vi "strain sensor program.vi"() -> ()   [LabVIEW 2016]
uses:
  Program Files (x86)/National Instruments/LabVIEW 2017/instr.lib/Keithley 2000/Keithley 2000.lvlib
  Program Files (x86)/National Instruments/LabVIEW 2017/instr.lib/Keithley 2000/Public/Configure/Configure 2 Wire Resistance.vi
  Program Files (x86)/National Instruments/LabVIEW 2017/instr.lib/Keithley 2000/Public/Configure/Configure DC Current.vi
  Program Files (x86)/National Instruments/LabVIEW 2017/instr.lib/Keithley 2000/Public/Configure/Configure AC Current.vi
  Program Files (x86)/National Instruments/LabVIEW 2017/instr.lib/Keithley 2000/Public/Configure/Configure DC Volts.vi
  Program Files (x86)/National Instruments/LabVIEW 2017/instr.lib/Keithley 2000/Public/Configure/Configure AC Volts.vi
  Program Files (x86)/National Instruments/LabVIEW 2017/instr.lib/Keithley 2000/Public/Configure/Configure 4 Wire Resistance.vi
  <vilib>/Utility/file.llb/Write To Spreadsheet File (DBL).vi
panel:
  out "point numbers 2":i32
  out "Measurement 2":dbl
  out "Units 2":string
  out "Speed(X) 2":i32
  out "Position(X) 2":i32
  out "XY 그래프 2":cluster{dbl[], dbl[]}(graph)
  in  "?":bool
  in  "?":u16(ring) items=["+X", "-X", "+Y", "-Y"]
  out "Units":string
  out "Measurement":dbl
  in  "Function (0: DC Volts)":u16(ring)=4 items=["DC Volts", "AC Volts", "DC Current", "AC Current", "2-Wire Resistance", "4-Wire Resistance"]
  in  "VISA resource name":refnum<visa-resource-name>="GPIB0::16::INSTR"
  out "XY 그래프":cluster{dbl[], dbl[]}(graph)
  in  "file path (dialog if empty)":path
  out "Position(X)":i32
  out "Speed(X)":i32
  in  "Start":bool
  out "point numbers":i32
  in  "?":bool
  in  "?":u16(ring) items=["X", "Y"]
  in  "Set Speed":i32
  out "Read Speed":u32
  in  "Drive Speed Number":u16(ring) items=["Drive Speed 1", "Drive Speed 2", "Drive Speed 3", "Drive Speed 4"]
  in  "Drive speed Set":bool
  in  "Drive Speed Number":u16(ring) items=["Drive Speed 1", "Drive Speed 2", "Drive Speed 3", "Drive Speed 4"]
  in  "Axis":u16(ring) items=["X", "Y"]
  out "Speed":u32=1000
  in  "Speed Set":bool
  in  "AXIS":u16(ring)=1 items=["X", "Y"]
  in  "SPEED(1~4)":string="1"
  in  "x - axis start point (cm)":dbl
  out "baud rate output":refnum<visa-resource-name>
  in  "x - axis increment(cm)":dbl
  in  "baud rate (9600)":u32=9600
  in  "Port set":refnum<visa-resource-name>="COM3"
  in  "x - axis end point (cm)":dbl=10.0
  in  "?":bool
  # "Motor Control"
  # "DRIVE SPEED READ"
  # "DRIVE SPEED SELECT"
  # "DRIVE SPEED SET"
  # "Plot : Ohm-cm"
  # "POSITION & SPEED READ"
  # "Multimeter"
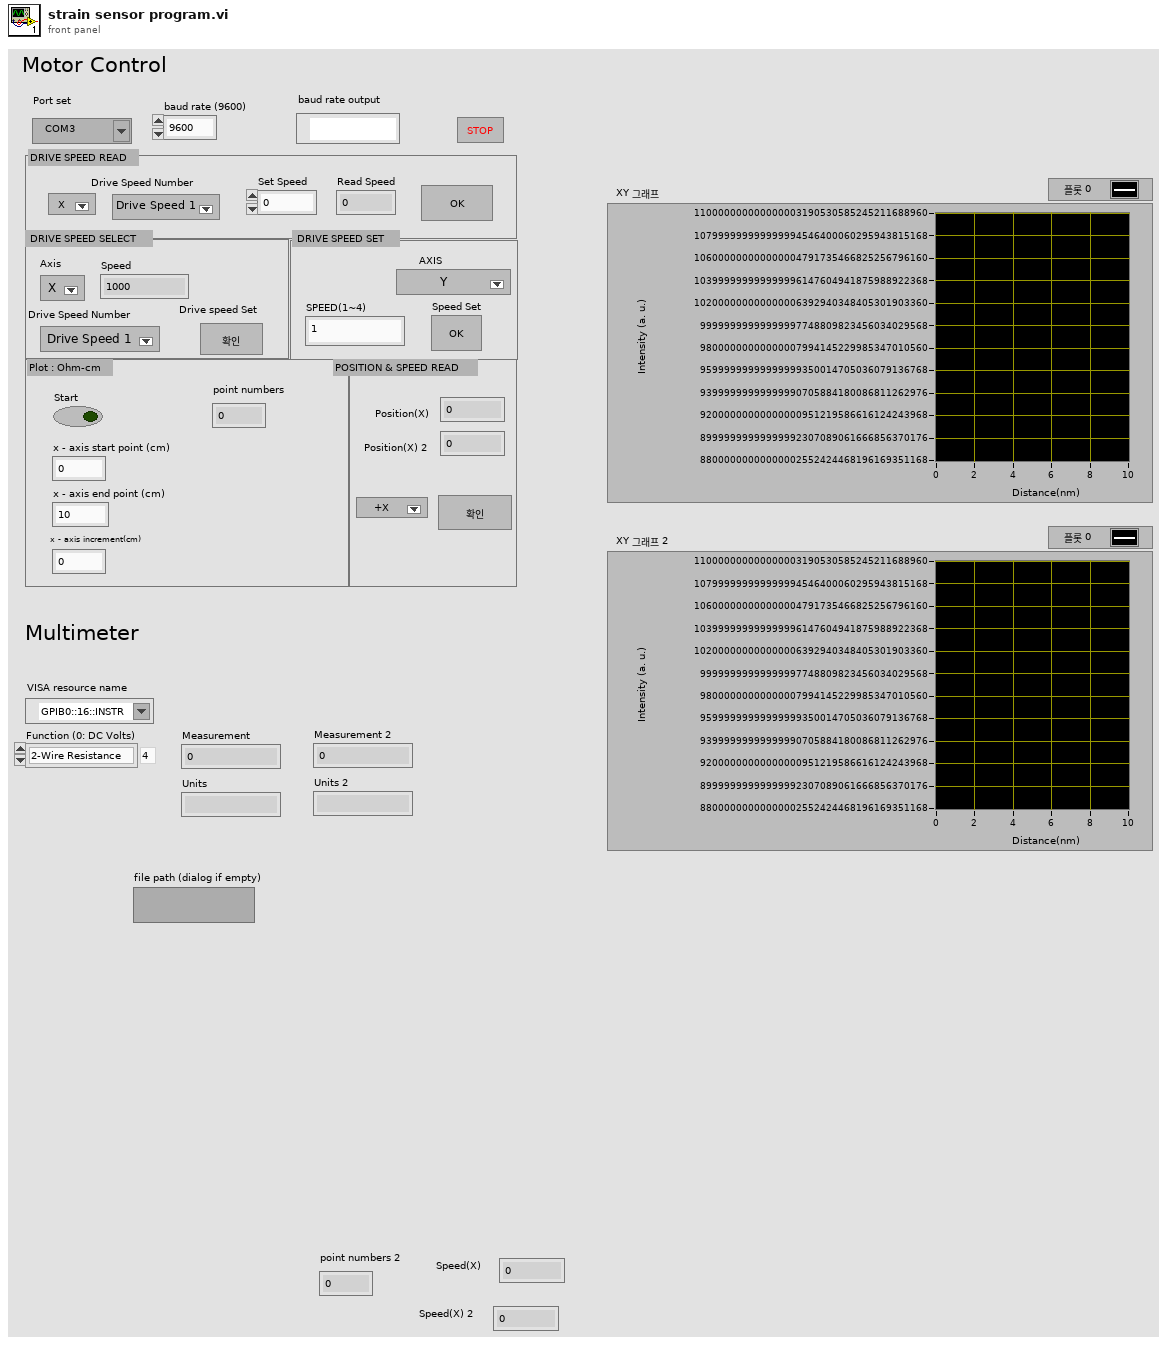
[diagram p1: front panel]
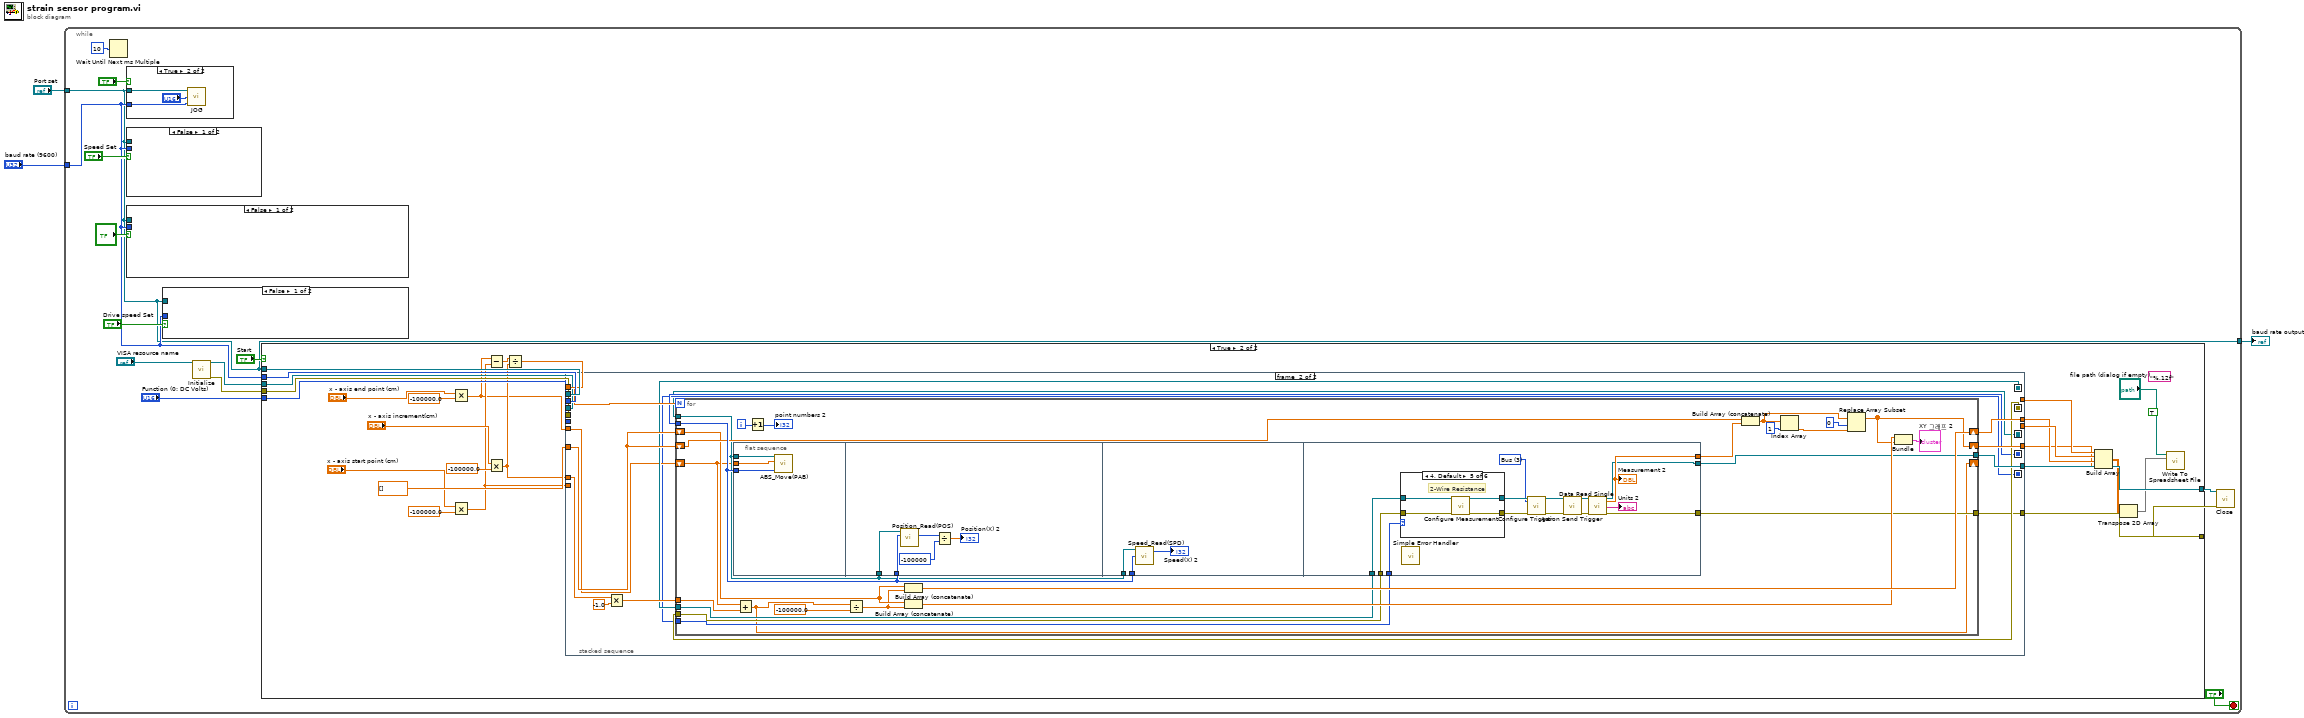
[diagram p0: block diagram]
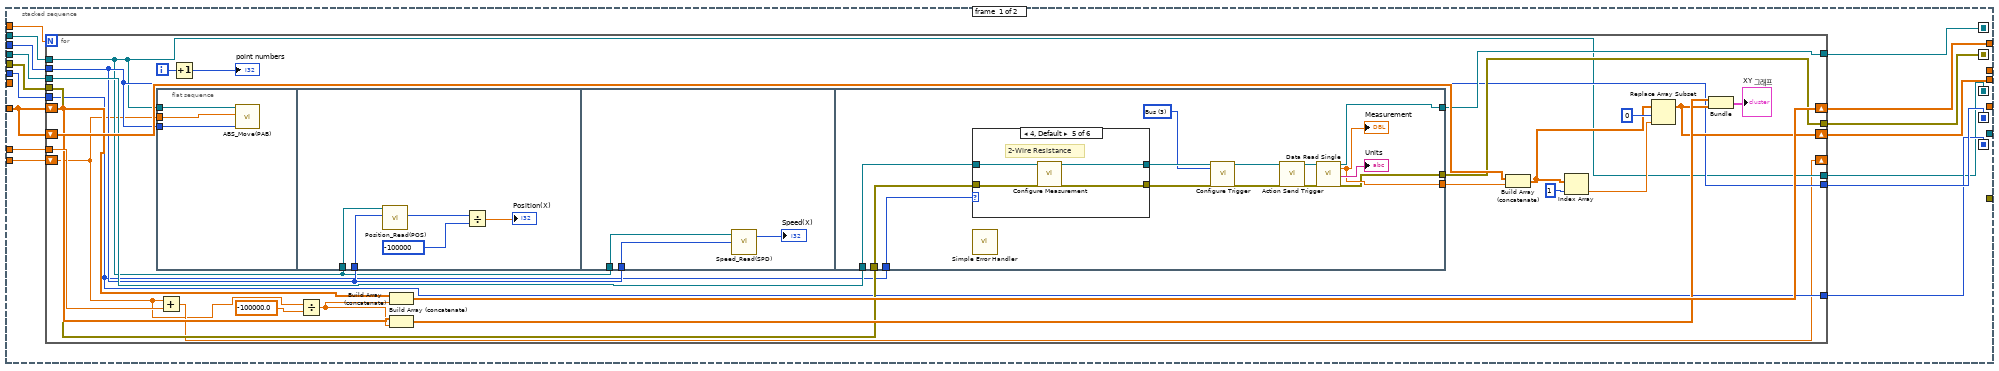
[diagram p4: hidden frame]
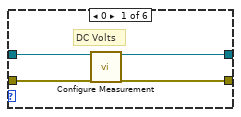
[diagram p5: hidden frame]
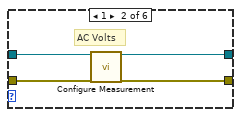
[diagram p6: hidden frame]
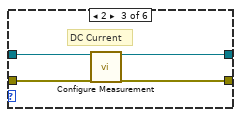
[diagram p7: hidden frame]
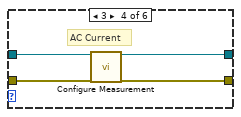
[diagram p8: hidden frame]
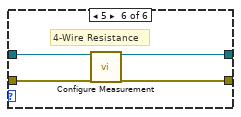
[diagram p9: hidden frame]
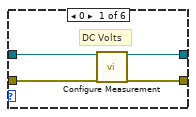
[diagram p10: hidden frame]
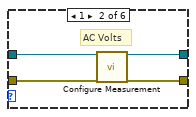
[diagram p11: hidden frame]
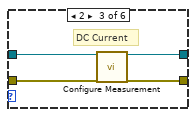
[diagram p12: hidden frame]
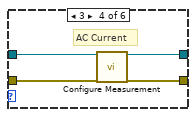
[diagram p13: hidden frame]
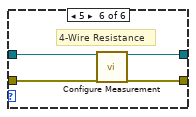
[diagram p14: hidden frame]
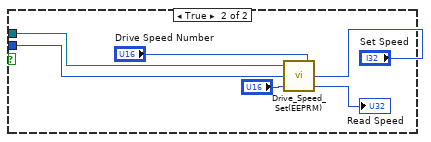
[diagram p15: hidden frame]
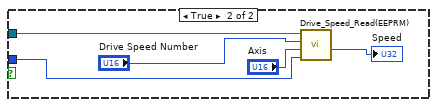
[diagram p16: hidden frame]
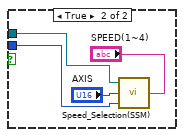
[diagram p17: hidden frame]
diagram:
  n1 = while {
    tunnel: "Port set" -> [w4]
    tunnel: "baud rate (9600)" -> [w5]
    tunnel: [w4] -> w1
    stop <- "?" stop-if-true
    n2 = Wait Until Next ms Multiple(millisecond multiple=u32 10 ("ms 배수")) -> ()  [unwired: 1 out]
    n3 = case shown="True" "?" {
      tunnel: w4 -> [_ w21]
      tunnel: w5 -> [_ w20]
      frame False {
      }
      frame True {
        n4 = call "JOG.vi"("baud rate (9600)"=w20, "AXIS"="?", "Port"=w21) -> ()  [unwired: 2 out]
      }
    }
    n5 = case shown="False" "Speed Set" {
      tunnel: w4 -> [_ w241]
      tunnel: w5 -> [_ w240]
      frame False {
      }
      frame True {
        n6 = call "Speed_Selection(SSM).vi"("SPEED(1~4)"="SPEED(1~4)", "baud rate (9600)"=w240, "AXIS"="AXIS", "Port"=w241) -> ()  [unwired: 2 out]
      }
    }
    n7 = case shown="False" "?" {
      tunnel: w4 -> [_ w232]
      tunnel: w5 -> [_ w227]
      frame False {
      }
      frame True {
        n8 = call "Drive_Speed_Set(EEPRM).vi"("Set Speed"="Set Speed", "Drive Speed Number"="Drive Speed Number", "Axis"="?", "baud rate (9600)"=w227, "Port"=w232) -> ("Read Speed"=→"Read Speed":u32)
      }
    }
    n9 = case shown="False" "Drive speed Set" {
      tunnel: w4 -> [_ w237]
      tunnel: w5 -> [_ w233]
      frame False {
      }
      frame True {
        n10 = call "Drive_Speed_Read(EEPRM).vi"("baud rate (9600)"=w233, "Axis"="Axis", "Drive Speed Number"="Drive Speed Number", "Port"=w237) -> ("Spped"=→"Speed":u32)  [unwired: 1 in, 3 out]
      }
    }
    n11 = call "Initialize.vi"("VISA resource name"="VISA resource name") -> ("VISA resource name out"=w10:refnum<visa-resource-name>, "error out"=w9:errorcluster)  [unwired: 17 in]
    n12 = case shown="True" "Start" {
      tunnel: w4 -> [_ w47]
      tunnel: w5 -> [_ w46]
      tunnel: "Function (0: DC Volts)" -> [_ w40]
      tunnel: w10 -> [_ w39]
      tunnel: w9 -> [_ w38]
      tunnel: [_ w37] -> w8
      tunnel: [_ w36] -> w7
      frame False {
      }
      frame True {
        (unwired) "%.12f" ("format (%.3f)")
        (unwired) TRUE
        n13 = Multiply(x="x - axis end point (cm)", y=-100000.0) -> (x*y=w27:dbl)
        n14 = Multiply(x="x - axis start point (cm)", y=-100000.0) -> (x*y=w28:dbl)
        n15 = Subtract(x=w27, y=w28) -> (x-y=w45:dbl)
        n16 = Multiply(x="x - axis increment(cm)", y=-100000.0) -> (x*y=w31:dbl)
        n17 = Divide(x=w45, y=w31) -> (x/y=w44:dbl)
        n18 = stacked-sequence {
          seq-local: [w52 _] -> [_ w144]
          seq-local: [w51 _] -> [_ w143]
          seq-local: [w50 _] -> [_ w140]
          seq-local: [w49 _] -> [_ w139]
          seq-local: [w48 _] -> [_ w138]
          tunnel: w47 -> [w63 _]
          tunnel: w46 -> [w62 _]
          tunnel: w44 -> [w61 w151]
          tunnel: dbl[] [] -> [w60 w152]
          tunnel: [w59 _] -> w42
          tunnel: [w58 _] -> w41
          tunnel: w40 -> [w57 _]
          tunnel: w39 -> [w56 _]
          tunnel: w38 -> [w55 _]
          tunnel: [_ w145] -> w37
          tunnel: [_ w142] -> w36
          tunnel: w31 -> [w54 w149]
          tunnel: w28 -> [w53 _]
          tunnel: [_ w147] -> w25
          tunnel: [_ w146] -> w24
          tunnel: w27 -> [_ w141]
          frame #0 {
            n19 = for {
              N: w61 -> [_]
              tunnel: w54 -> [w86]
              shift-right: [w65] -> _
              shift-left: w53 -> [w64]
              tunnel: w63 -> [w66]
              tunnel: w62 -> [w68]
              shift-right: [w84] -> w59
              shift-left: w60 -> [w81]
              shift-right: [w70] -> w58
              shift-left: w60 -> [w85]
              tunnel: w57 -> [w67]
              tunnel: w56 -> [w80]
              tunnel: w55 -> [w79]
              tunnel: [w78] -> w52
              tunnel: [w77] -> w51
              tunnel: [w68] -> w50
              tunnel: [w67] -> w49
              tunnel: [w66] -> w48
              i -> [w88]
              n20 = flat-sequence {
                tunnel: w68 -> [w91]
                tunnel: w66 -> [w90]
                tunnel: w64 -> [w89]
                tunnel: w68 -> [w96]
                tunnel: w66 -> [w95]
                tunnel: w68 -> [w98]
                tunnel: w66 -> [w97]
                tunnel: [w105] -> w82
                tunnel: w67 -> [w104]
                tunnel: w80 -> [w103]
                tunnel: w79 -> [w102]
                tunnel: [w101] -> w78
                tunnel: [w100] -> w77
                frame #0 {
                  n21 = call "ABS_Move(PAB).vi"("baud rate (9600)"=w91, "X Position(ABS)"=w89, "Port"=w90) -> ()  [unwired: 3 in, 3 out]
                }
                frame #1 {
                  n22 = call "Position_Read(POS).vi"("baud rate (9600)"=w96, "Port"=w95) -> ("Position(X)"=w93:i32)  [unwired: 2 in, 4 out]
                  n23 = Divide(x=w93, y=-100000) -> (x/y=→"Position(X)":dbl)
                }
                frame #2 {
                  n24 = call "Speed_Read(SPD).vi"("baud rate (9600)"=w98, "Port"=w97) -> ("Speed(X)"=→"Speed(X)":i32)  [unwired: 1 in, 2 out]
                }
                frame #3 {
                  w110 = u16 3 items=["Immediate", "Timer", "Manual", "Bus", "External"] ("Source (0: Immediate)")
                  n25 = case shown="4, Default" w104 {
                    tunnel: w102 -> [w117 w121 w125 w129 w133 w137]
                    tunnel: w103 -> [w116 w120 w124 w128 w132 w136]
                    tunnel: [w115 w119 w123 w127 w131 w135] -> w113
                    tunnel: [w114 w118 w122 w126 w130 w134] -> w112
                    frame 0 {
                      # "DC Volts"
                      n26 = call-poly "Configure Measurement.vi"("VISA resource name"=w116, "error in (no error)"=w117) -> ("VISA resource name out"=w114:refnum<visa-resource-name>, "error out"=w115:errorcluster)  [unwired: 16 in]
                    }
                    frame 1 {
                      # "AC Volts"
                      n27 = call-poly "Configure Measurement.vi"("VISA resource name"=w120, "error in (no error)"=w121) -> ("VISA resource name out"=w118:refnum<visa-resource-name>, "error out"=w119:errorcluster)  [unwired: 16 in]
                    }
                    frame 2 {
                      # "DC Current"
                      n28 = call-poly "Configure Measurement.vi"("VISA resource name"=w124, "error in (no error)"=w125) -> ("VISA resource name out"=w122:refnum<visa-resource-name>, "error out"=w123:errorcluster)  [unwired: 16 in]
                    }
                    frame 3 {
                      # "AC Current"
                      n29 = call-poly "Configure Measurement.vi"("VISA resource name"=w128, "error in (no error)"=w129) -> ("VISA resource name out"=w126:refnum<visa-resource-name>, "error out"=w127:errorcluster)  [unwired: 16 in]
                    }
                    frame 4, Default {
                      # "2-Wire Resistance"
                      n30 = call-poly "Configure Measurement.vi"("VISA resource name"=w132, "error in (no error)"=w133) -> ("VISA resource name out"=w130:refnum<visa-resource-name>, "error out"=w131:errorcluster)  [unwired: 16 in]
                    }
                    frame 5 {
                      # "4-Wire Resistance"
                      n31 = call-poly "Configure Measurement.vi"("VISA resource name"=w136, "error in (no error)"=w137) -> ("VISA resource name out"=w134:refnum<visa-resource-name>, "error out"=w135:errorcluster)  [unwired: 16 in]
                    }
                  }
                  n32 = call <vilib>:"Simple Error Handler.vi"() -> ()  [unwired: 5 in, 5 out]
                  n33 = call "Configure Trigger.vi"("VISA resource name"=w112, "Source (0: Immediate)"=w110, "error in (no error)"=w113) -> ("VISA resource name out"=w109:refnum<visa-resource-name>, "error out"=w108:errorcluster)  [unwired: 15 in]
                  n34 = call "Action Send Trigger.vi"("VISA resource name"=w109, "error in (no error)"=w108) -> ("VISA resource name out"=w106:refnum<visa-resource-name>, "error out"=w107:errorcluster)  [unwired: 16 in]
                  n35 = call "Data Read Single.vi"("VISA resource name"=w106, "error in (no error)"=w107) -> ("VISA resource name out"=w101:refnum<visa-resource-name>, "Measurement"=w105:dbl, "Units"=→"Units":string, "error out"=w100:errorcluster)  [unwired: 13 in, 1 out]
                  "Measurement" <- w105
                }
              }
              n36 = Add(x=w64, y=w86) -> (x+y=w65:dbl)
              n37 = Increment(x=w88) -> (x+1=→"point numbers":i32)
              n38 = Divide(x=w64, y=-100000.0) -> (x/y=w72:dbl)
              n39 = Build Array (concatenate)(w81, w72) -> (w84:dbl[])
              n40 = Build Array (concatenate)(w81, w72) -> (w83:dbl[])
              n41 = Build Array (concatenate)(w85, w82) -> (w71:dbl[])
              n42 = Index Array(array=w71, index=1) -> (element=w74:dbl)
              n43 = Replace Array Subset(array=w71, new element=w74, index=0) -> (w70:dbl[])
              n44 = Bundle(w83, w70) -> (→"XY 그래프":cluster{dbl[], dbl[]})  [unwired: 1 in]
            }
          }
          frame #1 {
            n45 = Multiply(x=w149, y=-1.0) -> (x*y=w148:dbl)
            n46 = for {
              N: w151 -> [_]
              tunnel: w148 -> [w174]
              shift-right: [w158] -> _
              shift-left: w141 -> [w153]
              tunnel: w138 -> [w154]
              tunnel: w140 -> [w175]
              shift-right: [w172] -> w147
              shift-left: w152 -> [w169]
              shift-right: [w156] -> w146
              shift-left: w152 -> [w173]
              tunnel: w139 -> [w168]
              tunnel: w144 -> [w167]
              tunnel: w143 -> [w166]
              tunnel: [w165] -> w145
              tunnel: [w164] -> w142
              i -> [w177]
              n47 = flat-sequence {
                tunnel: w175 -> [w180]
                tunnel: w154 -> [w179]
                tunnel: w153 -> [w178]
                tunnel: w175 -> [w185]
                tunnel: w154 -> [w184]
                tunnel: w175 -> [w187]
                tunnel: w154 -> [w186]
                tunnel: [w194] -> w170
                tunnel: w168 -> [w193]
                tunnel: w167 -> [w192]
                tunnel: w166 -> [w191]
                tunnel: [w190] -> w165
                tunnel: [w189] -> w164
                frame #0 {
                  n48 = call "ABS_Move(PAB).vi"("baud rate (9600)"=w180, "X Position(ABS)"=w178, "Port"=w179) -> ()  [unwired: 3 in, 3 out]
                }
                frame #1 {
                  n49 = call "Position_Read(POS).vi"("baud rate (9600)"=w185, "Port"=w184) -> ("Position(X)"=w182:i32)  [unwired: 2 in, 4 out]
                  n50 = Divide(x=w182, y=-100000) -> (x/y=→"Position(X) 2":dbl)
                }
                frame #2 {
                  n51 = call "Speed_Read(SPD).vi"("baud rate (9600)"=w187, "Port"=w186) -> ("Speed(X)"=→"Speed(X) 2":i32)  [unwired: 1 in, 2 out]
                }
                frame #3 {
                  w199 = u16 3 items=["Immediate", "Timer", "Manual", "Bus", "External"] ("Source (0: Immediate)")
                  n52 = case shown="4, Default" w193 {
                    tunnel: w191 -> [w206 w210 w214 w218 w222 w226]
                    tunnel: w192 -> [w205 w209 w213 w217 w221 w225]
                    tunnel: [w204 w208 w212 w216 w220 w224] -> w202
                    tunnel: [w203 w207 w211 w215 w219 w223] -> w201
                    frame 0 {
                      # "DC Volts"
                      n53 = call-poly "Configure Measurement.vi"("VISA resource name"=w205, "error in (no error)"=w206) -> ("VISA resource name out"=w203:refnum<visa-resource-name>, "error out"=w204:errorcluster)  [unwired: 16 in]
                    }
                    frame 1 {
                      # "AC Volts"
                      n54 = call-poly "Configure Measurement.vi"("VISA resource name"=w209, "error in (no error)"=w210) -> ("VISA resource name out"=w207:refnum<visa-resource-name>, "error out"=w208:errorcluster)  [unwired: 16 in]
                    }
                    frame 2 {
                      # "DC Current"
                      n55 = call-poly "Configure Measurement.vi"("VISA resource name"=w213, "error in (no error)"=w214) -> ("VISA resource name out"=w211:refnum<visa-resource-name>, "error out"=w212:errorcluster)  [unwired: 16 in]
                    }
                    frame 3 {
                      # "AC Current"
                      n56 = call-poly "Configure Measurement.vi"("VISA resource name"=w217, "error in (no error)"=w218) -> ("VISA resource name out"=w215:refnum<visa-resource-name>, "error out"=w216:errorcluster)  [unwired: 16 in]
                    }
                    frame 4, Default {
                      # "2-Wire Resistance"
                      n57 = call-poly "Configure Measurement.vi"("VISA resource name"=w221, "error in (no error)"=w222) -> ("VISA resource name out"=w219:refnum<visa-resource-name>, "error out"=w220:errorcluster)  [unwired: 16 in]
                    }
                    frame 5 {
                      # "4-Wire Resistance"
                      n58 = call-poly "Configure Measurement.vi"("VISA resource name"=w225, "error in (no error)"=w226) -> ("VISA resource name out"=w223:refnum<visa-resource-name>, "error out"=w224:errorcluster)  [unwired: 16 in]
                    }
                  }
                  n59 = call <vilib>:"Simple Error Handler.vi"() -> ()  [unwired: 5 in, 5 out]
                  n60 = call "Configure Trigger.vi"("VISA resource name"=w201, "Source (0: Immediate)"=w199, "error in (no error)"=w202) -> ("VISA resource name out"=w198:refnum<visa-resource-name>, "error out"=w197:errorcluster)  [unwired: 15 in]
                  n61 = call "Action Send Trigger.vi"("VISA resource name"=w198, "error in (no error)"=w197) -> ("VISA resource name out"=w195:refnum<visa-resource-name>, "error out"=w196:errorcluster)  [unwired: 16 in]
                  n62 = call "Data Read Single.vi"("VISA resource name"=w195, "error in (no error)"=w196) -> ("VISA resource name out"=w190:refnum<visa-resource-name>, "Measurement"=w194:dbl, "Units"=→"Units 2":string, "error out"=w189:errorcluster)  [unwired: 13 in, 1 out]
                  "Measurement 2" <- w194
                }
              }
              n63 = Add(x=w153, y=w174) -> (x+y=w158:dbl)
              n64 = Increment(x=w177) -> (x+1=→"point numbers 2":i32)
              n65 = Divide(x=w158, y=-100000.0) -> (x/y=w159:dbl)
              n66 = Build Array (concatenate)(w169, w159) -> (w172:dbl[])
              n67 = Build Array (concatenate)(w169, w159) -> (w171:dbl[])
              n68 = Build Array (concatenate)(w173, w170) -> (w157:dbl[])
              n69 = Index Array(array=w157, index=1) -> (element=w161:dbl)
              n70 = Replace Array Subset(array=w157, new element=w161, index=0) -> (w156:dbl[])
              n71 = Bundle(w171, w156) -> (→"XY 그래프 2":cluster{dbl[], dbl[]})  [unwired: 1 in]
            }
          }
        }
        n72 = Build Array(w42, w41, w25, w24) -> (w23:dbl[][])
        n73 = Transpose 2D Array(2D array=w23) -> (transposed array=w22:dbl[][])
        n74 = call-poly <vilib>:"Write To Spreadsheet File.vi"("2D data"=w22, "file path (dialog if empty)"="file path (dialog if empty)") -> ()  [unwired: 4 in, 3 out]
      }
    }
    n75 = call "Close.vi"("VISA resource name"=w8, "error in (no error)"=w7) -> ()  [unwired: 17 in, 1 out]
  }
  "baud rate output" <- w1
